vi "FGV-JKISM Modules.vi"(6 "Enum":T1, 7 "Module Name":string, 8 "Error in":errorcluster caption="Error in (no error)", 11 "Message":string) -> (0 "Error out":errorcluster, 3 "JKISM External Event":refnum<user-event>)   [LabVIEW 2017, in "_jkism_magic.lvlib"]
uses:
  _jkism_magic.lvlib
  _action.ctl
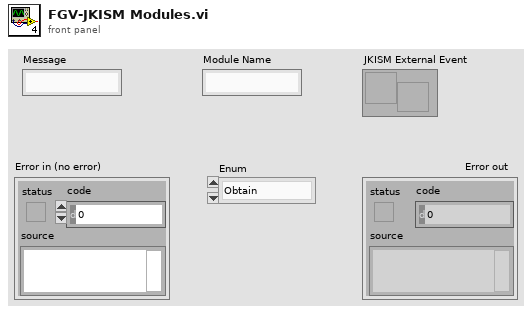
[diagram p1: front panel]
types:
  T1 = typedef "_jkism_magic.lvlib/_action.ctl" = enum16{"Obtain", "Destroy", "Broadcast", "Post"}
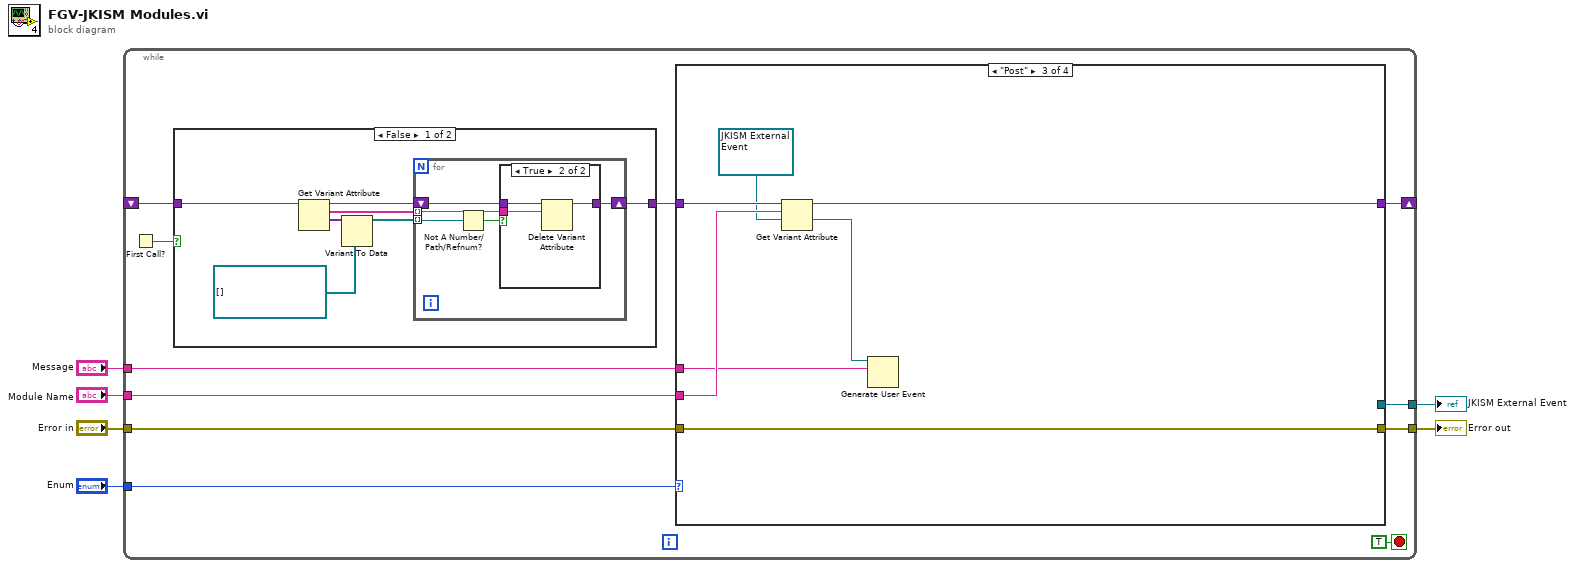
[diagram p0: block diagram]
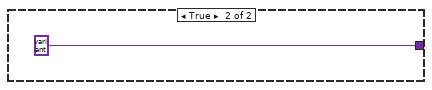
[diagram p3: hidden frame]
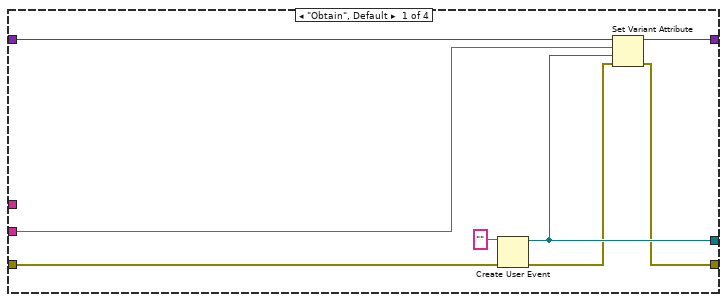
[diagram p4: hidden frame]
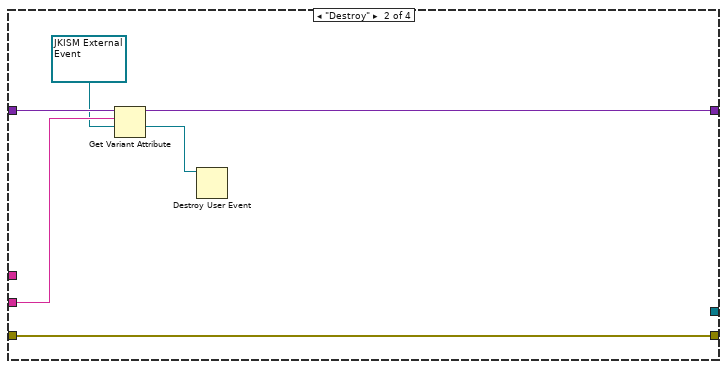
[diagram p5: hidden frame]
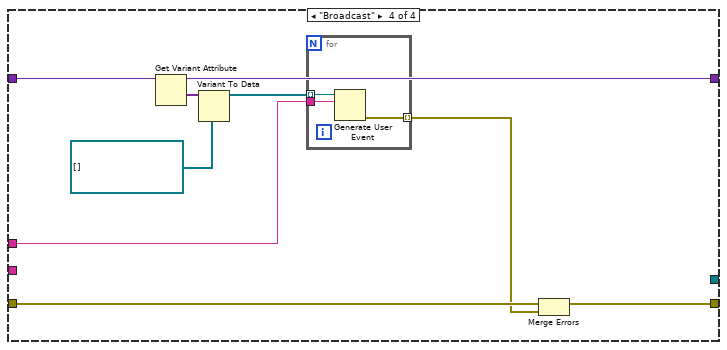
[diagram p6: hidden frame]
diagram:
  n1 = while {
    tunnel: [w16] -> w6
    tunnel: [w15] -> w5
    tunnel: "Error in" -> [w14]
    tunnel: "Enum" -> [w13]
    shift-right: [w12] -> _
    shift-left: _ -> [w10]
    tunnel: "Module Name" -> [w8]
    tunnel: "Message" -> [w7]
    stop <- TRUE stop-if-true
    n2 = First Call?() -> (First Call?: T/F=w9:bool)
    n3 = case shown="False" w9 {
      tunnel: [w23 variant] -> w11
      tunnel: w10 -> [w24 _]
      frame False {
        n4 = Get Variant Attribute(Variant=w24) -> (duplicate Variant=w22:variant, names=w21:string[], values=w20:variant[])  [unwired: 3 in, 1 out]
        n5 = Variant To Data(type=refnum<user-event>[] [], Variant=w20) -> (data=w18:refnum<user-event>[])  [unwired: 1 in, 1 out]
        n6 = for {
          shift-right: [w28] -> w23
          shift-left: w22 -> [w29]
          tunnel: w21 -> [w27] mode=indexing
          tunnel: w18 -> [w26] mode=indexing
          n7 = Not A Number/Path/Refnum?(number/path/refnum=w26) -> (NaN/Path/Refnum?=w25:bool)
          n8 = case shown="True" w25 {
            tunnel: w29 -> [w30 w33]
            tunnel: [w30 w32] -> w28
            tunnel: w27 -> [_ w31]
            frame False {
            }
            frame True {
              n9 = Delete Variant Attribute(6:w31, 7:w33) -> (3:w32:variant)  [unwired: 1 in, 2 out]
            }
          }
        }
      }
      frame True {
      }
    }
    n10 = case shown="\"Post\"" w13 {
      tunnel: [w37 _ _ _] -> w16
      tunnel: [w35 w47 w54 w57] -> w15
      tunnel: w14 -> [w41 w47 w54 w64]
      tunnel: [w39 w46 w53 w60] -> w12
      tunnel: w11 -> [w40 w48 w55 w61]
      tunnel: w8 -> [w38 w45 w52 _]
      tunnel: w7 -> [_ _ w49 w58]
      frame "Obtain", Default {
        n11 = Create User Event(user event datatype="" ("JKISM External Event"), error in=w41) -> (user event=w37:refnum<user-event>, error out=w36:errorcluster)
        n12 = Set Variant Attribute(Variant=w40, name=w38, value=w37, error in=w36) -> (Variant out=w39:variant, error out=w35:errorcluster)  [unwired: 1 out]
      }
      frame "Destroy" {
        n13 = Get Variant Attribute(Variant=w48, name=w45, default value (empty Variant)=refnum<user-event> refnum ("user event out")) -> (duplicate Variant=w46:variant, value=w43:refnum<user-event>)  [unwired: 1 in, 2 out]
        n14 = Destroy User Event(user event=w43) -> ()  [unwired: 1 in, 1 out]
      }
      frame "Post" {
        n15 = Get Variant Attribute(Variant=w55, name=w52, default value (empty Variant)=refnum<user-event> refnum ("user event out")) -> (duplicate Variant=w53:variant, value=w50:refnum<user-event>)  [unwired: 1 in, 2 out]
        n16 = Generate User Event(user event=w50, event data cluster=w49) -> ()  [unwired: 2 in, 2 out]
      }
      frame "Broadcast" {
        n17 = Get Variant Attribute(Variant=w61) -> (duplicate Variant=w60:variant, values=w62:variant[])  [unwired: 3 in, 2 out]
        n18 = Variant To Data(type=refnum<user-event>[] [], Variant=w62) -> (data=w59:refnum<user-event>[])  [unwired: 1 in, 1 out]
        n19 = for {
          tunnel: w59 -> [w67] mode=indexing
          tunnel: w58 -> [w66]
          tunnel: [w65] -> w56 mode=indexing
          n20 = Generate User Event(user event=w67, event data cluster=w66) -> (error out=w65:errorcluster)  [unwired: 2 in, 1 out]
        }
        n21 = Merge Errors(w64, w56) -> (w57:errorcluster)
      }
    }
  }
  "Error out" <- w5
  "JKISM External Event" <- w6
